vi "Record system names.vi"(0 "System(0)":u16, 1 "Action(GET)":enum16{"GET", "SET/Init"}(ring), 7 "Loop(0)":u16, 11 "error in (no error)":errorcluster, 12 "System type":variant, 13 "System Loops":variant[](array[variant])) -> (4 "System navn":string, 6 "Numb systems":i32, 8 "Loop name":string, 10 "Numb Loops in system":i32, 15 "error out":errorcluster)   [LabVIEW 2011]
uses:
  <vilib>/Utility/VariantDataType/GetNumericInfo.vi
  <vilib>/Utility/VariantDataType/VariantType.lvlib
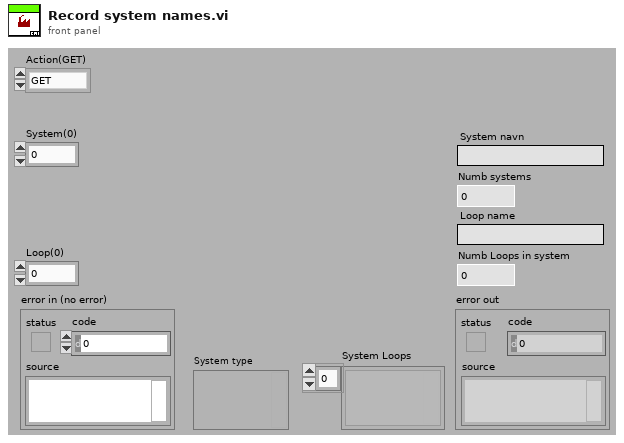
[diagram p1: front panel]
types:
  T1 = typedef "VariantType.lvlib/Type.ctl" = enum8{"Invalid Type", "Void", "I8", "I16", "I32", "I64", "U8", "U16", "U32", "U64", "Single Float", "Double Float", "Extended Float", "Single Complex", "Double Complex", "Extended Complex", "Enum U8", "Enum U16", "Enum U32", "Enum U64", "Single Float With Unit", "Double Float With Unit", "Extended Float With Unit", "Single Complex with Unit", "Double Complex with Unit", "Extended Complex with Unit", "Boolean", "String", "Path", "Picture", "Tag", "Array", "Cluster", "Variant", "LV Variant", "Waveform", "Timestamp", "Digital Waveform", "Digital Data", "ExpressData", "Refnum", "External Data", "VI", "Poly VI", "LabVIEW Class Instance", "Fixed Point"}
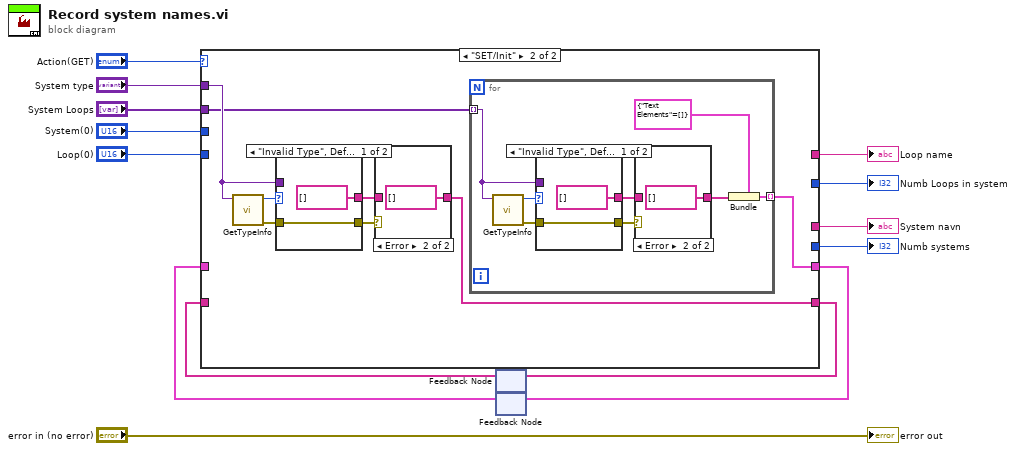
[diagram p0: block diagram]
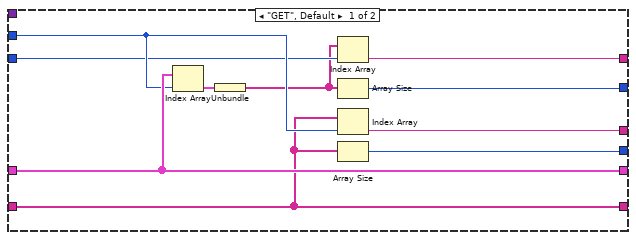
[diagram p2: hidden frame]
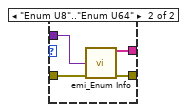
[diagram p4: hidden frame]
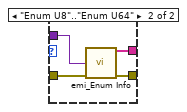
[diagram p6: hidden frame]
diagram:
  n1 = feedback #1() -> (w5:string[])  [unwired: 1 in]
  n2 = feedback #2() -> (w6:cluster{"Text Elements":string[]}[])  [unwired: 1 in]
  n3 = case shown="\"SET/Init\"" "Action(GET)" {
    tunnel: [w23 w25] -> w12
    tunnel: w6 -> [w23 _]
    tunnel: "System type" -> [_ w30]
    tunnel: "System Loops" -> [_ w26]
    tunnel: "System(0)" -> [w22 _]
    tunnel: "Loop(0)" -> [w20 _]
    tunnel: [w16 w27] -> w7
    tunnel: w5 -> [w16 _]
    tunnel: [w24 _] -> w4
    tunnel: [w19 _] -> w3
    tunnel: [w17 _] -> w2
    tunnel: [w15 _] -> w1
    frame "GET", Default {
      n4 = Index Array(array=w23, index=w22) -> (element=w21:cluster{"Text Elements":string[]})
      n5 = Unbundle(w21) -> ("Text Elements"=w18:string[])
      n6 = Index Array(array=w18, index=w20) -> (element=w19:string)
      n7 = Array Size(array=w18) -> (size(s)=w17:i32)
      n8 = Index Array(array=w16, index=w22) -> (element=w24:string)
      n9 = Array Size(array=w16) -> (size(s)=w15:i32)
    }
    frame "SET/Init" {
      n10 = call <vilib>:"GetTypeInfo.vi"("Variant"=w30) -> ("error out"=w31:errorcluster, "Type Enum"=w32:T1)  [unwired: 6 in, 3 out]
      n11 = case shown="\"Invalid Type\", Default" w32 {
        tunnel: w30 -> [_ w56]
        tunnel: w31 -> [w51 w55]
        tunnel: [string[] [] ("Text Elements") w54] -> w28
        tunnel: [w51 w53] -> w29
        frame "Invalid Type", Default {
        }
        frame "Enum U8".."Enum U64" {
          n12 = call "emi_Enum Info.vi"("Enum"=w56, "error in (no error)"=w55) -> ("Text Elements"=w54:string[], "error out"=w53:errorcluster)  [unwired: 10 in, 2 out]
        }
      }
      n13 = case shown="Error" w29 {
        tunnel: [w49 string[] [] ("Text Elements")] -> w27
        tunnel: w28 -> [w49 _]
        frame No Error {
        }
        frame Error {
        }
      }
      n14 = for {
        tunnel: w26 -> [w36] mode=indexing
        tunnel: [w33] -> w25 mode=indexing
        n15 = call <vilib>:"GetTypeInfo.vi"("Variant"=w36) -> ("error out"=w38:errorcluster, "Type Enum"=w37:T1)  [unwired: 6 in, 3 out]
        n16 = case shown="\"Invalid Type\", Default" w37 {
          tunnel: w36 -> [_ w48]
          tunnel: w38 -> [w43 w47]
          tunnel: [string[] [] ("Text Elements") w46] -> w40
          tunnel: [w43 w45] -> w39
          frame "Invalid Type", Default {
          }
          frame "Enum U8".."Enum U64" {
            n17 = call "emi_Enum Info.vi"("Enum"=w48, "error in (no error)"=w47) -> ("Text Elements"=w46:string[], "error out"=w45:errorcluster)  [unwired: 10 in, 2 out]
          }
        }
        n18 = case shown="Error" w39 {
          tunnel: [w41 string[] [] ("Text Elements")] -> w35
          tunnel: w40 -> [w41 _]
          frame No Error {
          }
          frame Error {
          }
        }
        n19 = Bundle(cluster=cluster{"Text Elements":string[]} {"Text Elements"=[]} ("output cluster"), "Text Elements"=w35) -> (w33:cluster{"Text Elements":string[]})
      }
    }
  }
  "System navn" <- w4
  "Loop name" <- w3
  "Numb Loops in system" <- w2
  "Numb systems" <- w1
  n20 = feedback-in #1(w7) -> ()
  n21 = feedback-in #2(w12) -> ()
  "error out" <- "error in (no error)"
